vi "PLL Lock.vi"(8 "error in (no error)":errorcluster, 10 "PLL lock  (T: Enable)":bool=TRUE, 11 "VISA resource name":refnum<visa-resource-name>) -> (0 "error out":errorcluster, 3 "VISA resource name out":refnum<visa-resource-name>)   [LabVIEW 2013, in "AWG.lvlib" / "Agilent 33XXX Series.lvlib"]
doc: "Enables or disables phase lock to 10 MHz reference input."
uses:
  Agilent 33XXX Series.lvlib
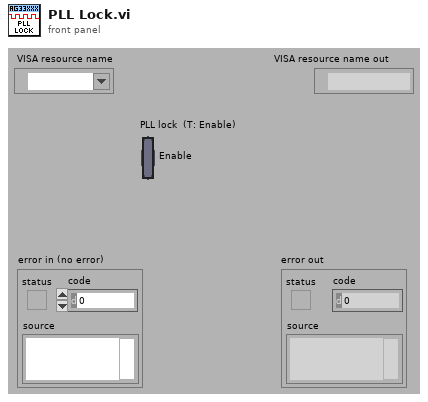
[diagram p1: front panel]
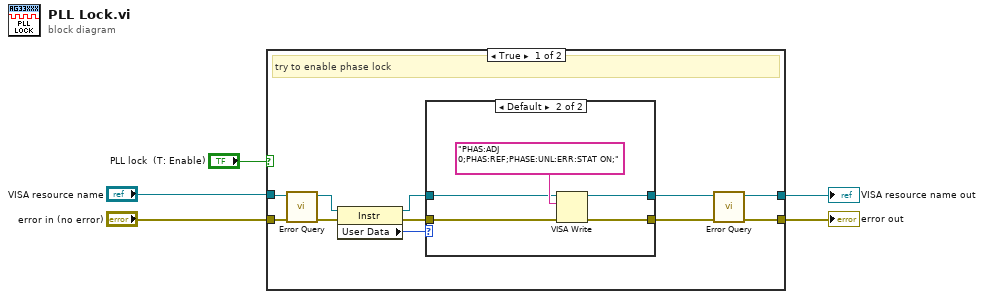
[diagram p0: block diagram]
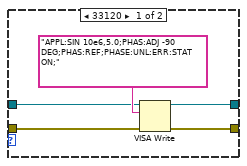
[diagram p2: hidden frame]
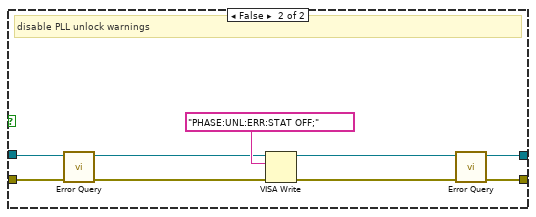
[diagram p3: hidden frame]
diagram:
  n1 = case shown="True" "PLL lock  (T: Enable)" {
    tunnel: [w14 w33] -> w4
    tunnel: [w13 w32] -> w5
    tunnel: "VISA resource name" -> [w11 w29]
    tunnel: "error in (no error)" -> [w12 w30]
    frame True {
      # "try to enable phase lock"
      n2 = call "Error Query.vi"("error in (no error)"=w12, "VISA resource name"=w11) -> ("error out"=w10:errorcluster, "VISA resource name out"=w9:refnum<visa-resource-name>)  [unwired: 6 in, 2 out]
      n3 = property class="Instr"(reference=w9, error in=w10) -> (reference out=w7:refnum<visa-resource-name>, error out=w8:errorcluster, "User Data"=w6:u32)
      n4 = case shown="Default" w6 {
        tunnel: [w21 w26] -> w16
        tunnel: [w20 w25] -> w15
        tunnel: w7 -> [w18 w23]
        tunnel: w8 -> [w17 w22]
        frame 33120 {
          n5 = VISA Write(VISA resource name=w18, write buffer="APPL:SIN 10e6,5.0;PHAS:ADJ -90 DEG;PHAS:REF;PHASE:UNL:ERR:STAT ON;", error in (no error)=w17) -> (VISA resource name out=w20:refnum<visa-resource-name>, error out=w21:errorcluster)  [unwired: 1 out]
        }
        frame Default {
          n6 = VISA Write(VISA resource name=w23, write buffer="PHAS:ADJ 0;PHAS:REF;PHASE:UNL:ERR:STAT ON;", error in (no error)=w22) -> (VISA resource name out=w25:refnum<visa-resource-name>, error out=w26:errorcluster)  [unwired: 1 out]
        }
      }
      n7 = call "Error Query.vi"("error in (no error)"=w16, "VISA resource name"=w15) -> ("error out"=w13:errorcluster, "VISA resource name out"=w14:refnum<visa-resource-name>)  [unwired: 6 in, 2 out]
    }
    frame False {
      # "disable PLL unlock warnings"
      n8 = call "Error Query.vi"("error in (no error)"=w30, "VISA resource name"=w29) -> ("error out"=w27:errorcluster, "VISA resource name out"=w28:refnum<visa-resource-name>)  [unwired: 6 in, 2 out]
      n9 = VISA Write(VISA resource name=w28, write buffer="PHASE:UNL:ERR:STAT OFF;", error in (no error)=w27) -> (VISA resource name out=w34:refnum<visa-resource-name>, error out=w35:errorcluster)  [unwired: 1 out]
      n10 = call "Error Query.vi"("error in (no error)"=w35, "VISA resource name"=w34) -> ("error out"=w32:errorcluster, "VISA resource name out"=w33:refnum<visa-resource-name>)  [unwired: 6 in, 2 out]
    }
  }
  "error out" <- w5
  "VISA resource name out" <- w4
